vi "File_DeleteElement.vi"(1 "Filepath":path, 3 "Recursive?":bool=TRUE, 5 "error in (no error)":errorcluster) -> (19 "error out":errorcluster)   [LabVIEW 2016]
doc: "Deletes a file or folder. Works on LLB as well. If folder, delete is performed recursively."
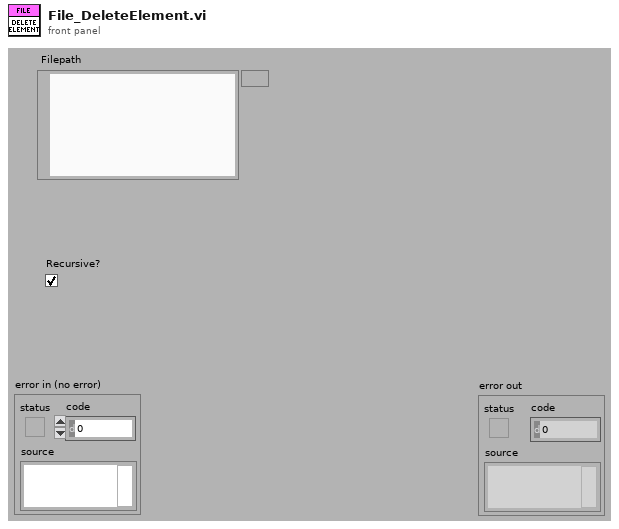
[diagram p1: front panel]
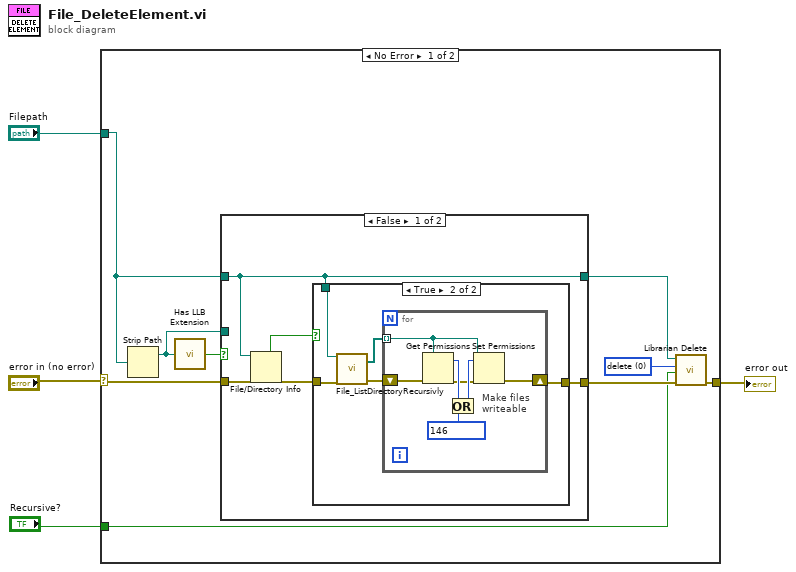
[diagram p0: block diagram]
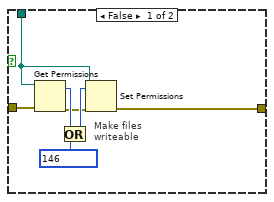
[diagram p2: hidden frame]
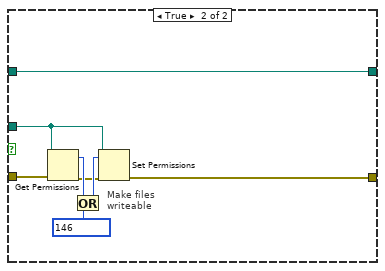
[diagram p3: hidden frame]
diagram:
  n1 = case shown="No Error" "error in (no error)" {
    selector: "error in (no error)" -> [w13 w46]
    tunnel: "Filepath" -> [w6 _]
    tunnel: [w10 w46] -> w2
    tunnel: "Recursive?" -> [w7 _]
    frame No Error {
      w8 = u16 0 items=["delete", "ask first"] ("delete")
      n2 = Strip Path(path=w6) -> (stripped path=w5:path)  [unwired: 1 out]
      n3 = call <vilib>:"Has LLB Extension.vi"("path"=w5) -> ("path to VI library?"=w12:bool)
      n4 = case shown="False" w12 {
        tunnel: [w18 w45] -> w11
        tunnel: [w15 w39] -> w9
        tunnel: w13 -> [w16 w40]
        tunnel: w6 -> [w15 w39]
        tunnel: w5 -> [_ w38]
        frame False {
          n5 = File/Directory Info(path=w15, error in=w16) -> (directory=w14:bool, error out=w17:errorcluster)  [unwired: 5 out]
          n6 = case shown="True" w14 {
            tunnel: [w25 w28] -> w18
            tunnel: w17 -> [w20 w30]
            tunnel: w15 -> [w19 w29]
            frame False {
              # "Make files\nwriteable"
              n7 = Get Permissions(8:w20, 11:w19) -> (0:w21:errorcluster, 5:w22:i16)  [unwired: 3 out]
              n8 = Or(x=w22, y=i16 146) -> (x .or. y?=w23:i16)
              n9 = Set Permissions(7:w23, 8:w21, 11:w19) -> (0:w25:errorcluster)  [unwired: 3 out]
            }
            frame True {
              n10 = call <resource>:"File_ListDirectoryRecursivly.vi"("DirPath"=w29, "error in (no error)"=w30) -> ("Files"=w26:path[], "error out"=w27:errorcluster)  [unwired: 2 in, 14 out]
              n11 = for {
                shift-right: [w33] -> w28
                shift-left: w27 -> [w32]
                tunnel: w26 -> [w31] mode=indexing
                # "Make files\nwriteable"
                n12 = Get Permissions(8:w32, 11:w31) -> (0:w34:errorcluster, 5:w35:i16)  [unwired: 3 out]
                n13 = Or(x=w35, y=i16 146) -> (x .or. y?=w36:i16)
                n14 = Set Permissions(7:w36, 8:w34, 11:w31) -> (0:w33:errorcluster)  [unwired: 3 out]
              }
            }
          }
        }
        frame True {
          # "Make files\nwriteable"
          n15 = Get Permissions(8:w40, 11:w38) -> (0:w41:errorcluster, 5:w42:i16)  [unwired: 3 out]
          n16 = Or(x=w42, y=i16 146) -> (x .or. y?=w43:i16)
          n17 = Set Permissions(7:w43, 8:w41, 11:w38) -> (0:w45:errorcluster)  [unwired: 3 out]
        }
      }
      n18 = call <vilib>:"Librarian Delete.vi"("error in (no error)"=w11, "recursive? (F)"=w7, "delete"=w8, "path"=w9) -> ("error out"=w10:errorcluster)  [unwired: 1 in, 6 out]
    }
    frame Error {
    }
  }
  "error out" <- w2
